vi "Write Message.vi"(8 "error in":errorcluster, 10 "message":string, 11 "Has Alarm in":refnum<class "Has Alarm.lvclass">) -> (0 "error out":errorcluster, 3 "Has Alarm out":refnum<class "Has Alarm.lvclass">)   [LabVIEW 2020, in "PV Access.lvlib" / "PV Data.lvlib" / "Has Alarm.lvclass"]
uses:
  Has Alarm.lvclass
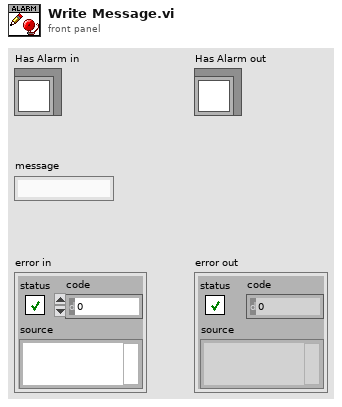
[diagram p1: front panel]
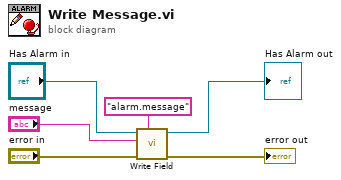
[diagram p0: block diagram]
diagram:
  n1 = call-dynamic "Write Field.vi"("field"="alarm.message", "error in (no error)"="error in", "value"="message", "Base Interface in"="Has Alarm in") -> ("error out"=→"error out":errorcluster, "Base Interface out"=→"Has Alarm out":refnum<class "Has Alarm.lvclass">)  [unwired: 6 in]
